vi "toStringArray.vi"(8 "error in (no error)":errorcluster, 11 "RampDown in":refnum<class "RampDown.lvclass">) -> (0 "error out":errorcluster, 2 "eventStringArray":string[](array[string]), 3 "RampDown out":refnum<class "RampDown.lvclass">)   [LabVIEW 2011, in "Tools.lvlib" / "Scripting.lvlib" / "RampDown.lvclass"]
uses:
  RampDown.lvclass
  RampEvent/RampEvent.lvclass
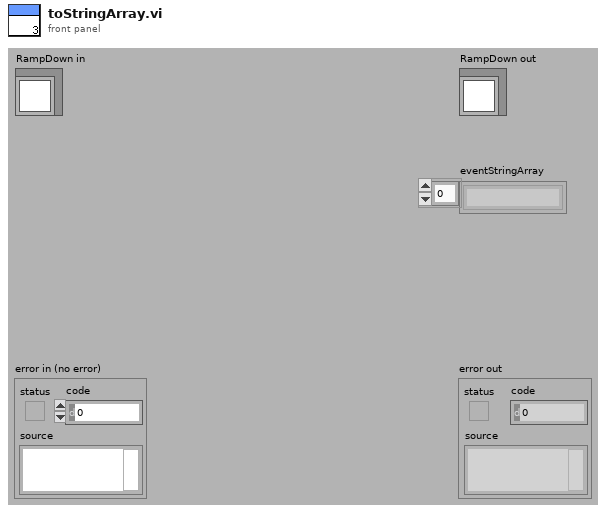
[diagram p1: front panel]
types:
  T1 = cluster{"rampTime":dbl, "timeStep":dbl, "dataValueStep":dbl}
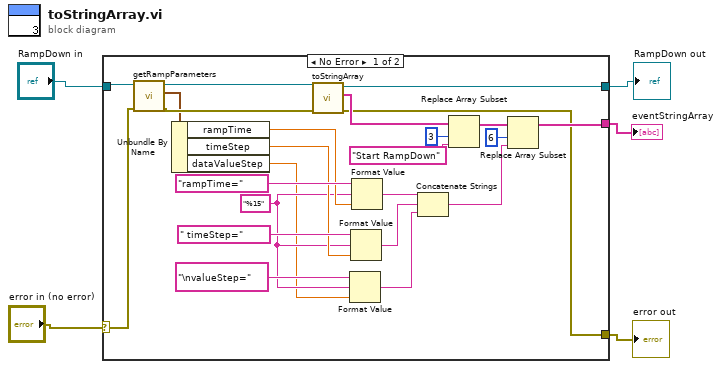
[diagram p0: block diagram]
diagram:
  n1 = case shown="No Error" "error in (no error)" {
    selector: "error in (no error)" -> [w8 w30]
    tunnel: "RampDown in" -> [w9 w31]
    tunnel: [w29 w31] -> w2
    tunnel: [w11 w30] -> w3
    tunnel: [w12 _] -> w1
    frame No Error {
      w23 = "%15"
      n2 = call "getRampParameters.vi"("error in (no error)"=w8, "RampEvent in"=w9) -> ("error out"=w7:errorcluster, "RampParameters"=w6:T1, "RampEvent out"=w10:refnum<class "RampDown.lvclass">)  [unwired: 7 in]
      n3 = Unbundle By Name(w6) -> ("rampTime"=w27:dbl, "timeStep"=w25:dbl, "dataValueStep"=w22:dbl)
      n4 = call-parent "toStringArray.vi"("error in (no error)"=w7, "RampEvent in"=w10) -> ("error out"=w11:errorcluster, "eventStringArray"=w21:string[], "RampEvent out"=w29:refnum<class "RampDown.lvclass">)  [unwired: 7 in]
      n5 = Format Value(string ("")="\nvalueStep=", format string=w23, value (0)=w22) -> (output string=w14:string)
      n6 = Format Value(string ("")=" timeStep=", format string=w23, value (0)=w25) -> (output string=w15:string)
      n7 = Format Value(string ("")="rampTime=", format string=w23, value (0)=w27) -> (output string=w16:string)
      n8 = Concatenate Strings(w16, w15, w14) -> (w13:string)
      n9 = Replace Array Subset(array=w21, new element="Start RampDown", index=3) -> (w19:string[])
      n10 = Replace Array Subset(array=w19, new element=w13, index=6) -> (w12:string[])
    }
    frame Error {
    }
  }
  "error out" <- w3
  "RampDown out" <- w2
  "eventStringArray" <- w1
